vi "Registerkarten ein-ausblenden.vi"(0 "Registerkartenreferenz":refnum<vi>, 11 "error in (no error)":errorcluster caption="Fehler (Eingang, kein Fehler)", 13 "Aktion":T1) -> (15 "error out":errorcluster caption="Fehler (Ausgang)")   [LabVIEW 2020, in "EPA 1065.lvlib"]
uses:
  EPA 1065.lvlib
  Aktion Registerkarten ein-ausblenden.ctl
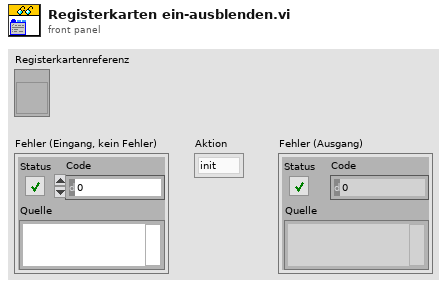
[diagram p1: front panel]
types:
  T1 = typedef "EPA 1065.lvlib/Aktion Registerkarten ein-ausblenden.ctl" = enum16{"init", "alle ausblenden", "Seite einblenden", "alle einblenden", "Seite deaktivieren", "Seiten aktivieren"}
  T2 = enum32{"Page Enabled", "Page Disabled", "Page Disabled & Grayed"}
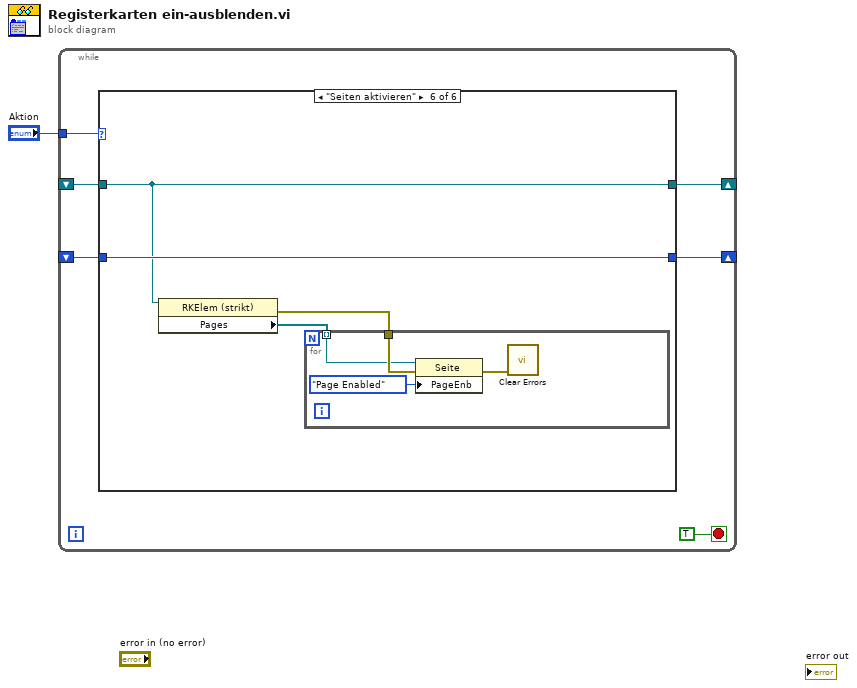
[diagram p0: block diagram]
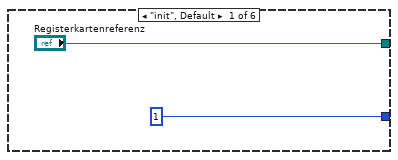
[diagram p2: hidden frame]
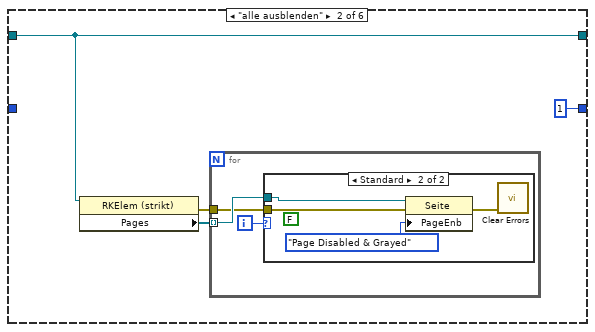
[diagram p3: hidden frame]
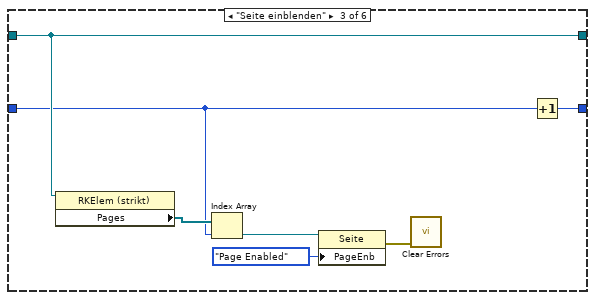
[diagram p5: hidden frame]
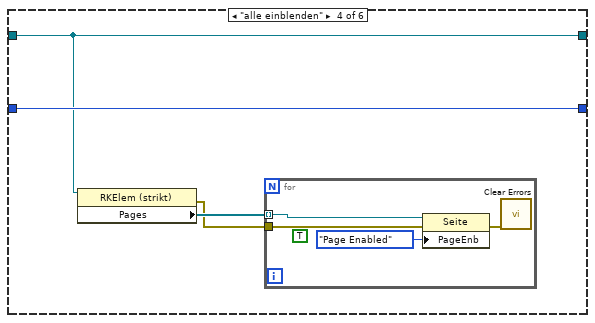
[diagram p6: hidden frame]
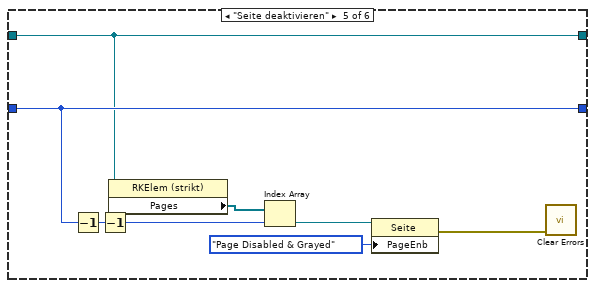
[diagram p7: hidden frame]
diagram:
  n1 = while {
    tunnel: "Aktion" -> [w7]
    shift-right: [w4] -> _
    shift-left: _ -> [w3]
    shift-right: [w5] -> _
    shift-left: _ -> [w2]
    stop <- TRUE stop-if-true
    n2 = case shown="\"Seiten aktivieren\"" w7 {
      tunnel: ["Registerkartenreferenz" w11 w26 w28 w38 w46] -> w5
      tunnel: [1 1 w27 w31 w43 w47] -> w4
      tunnel: w3 -> [_ _ w24 w31 w43 w47]
      tunnel: w2 -> [_ w11 w26 w28 w38 w46]
      frame "init", Default {
      }
      frame "alle ausblenden" {
        n3 = property class="RKElem (strikt)"(reference=w11) -> (error out=w12:errorcluster, "Pages"=w13:refnum<vi>[])  [unwired: 1 in, 1 out]
        n4 = for {
          tunnel: w13 -> [w16] mode=indexing
          tunnel: w12 -> [w14]
          i -> [w15]
          n5 = case shown="Standard" w15 {
            tunnel: w16 -> [_ w20]
            tunnel: w14 -> [_ w19]
            frame 0 {
            }
            frame Default {
              (unwired) FALSE ("Seite sichtbar")
              n6 = property class="Seite"(reference=w20, error in=w19, "PageEnb"=T2."Page Disabled & Grayed" ("Aktiv-Status der Seite")) -> (error out=w18:errorcluster)  [unwired: 1 out]
              n7 = call <vilib>:"Clear Errors.vi"("error in (no error)"=w18) -> ()  [unwired: 5 in, 2 out]
            }
          }
        }
      }
      frame "Seite einblenden" {
        n8 = property class="RKElem (strikt)"(reference=w26) -> ("Pages"=w25:refnum<vi>[])  [unwired: 1 in, 2 out]
        n9 = Index Array(array=w25, index=w24) -> (element=w21:refnum<vi>)
        n10 = property class="Seite"(reference=w21, "PageEnb"=T2."Page Enabled" ("Aktiv-Status der Seite")) -> (error out=w23:errorcluster)  [unwired: 1 in, 1 out]
        n11 = call <vilib>:"Clear Errors.vi"("error in (no error)"=w23) -> ()  [unwired: 5 in, 2 out]
        n12 = Increment(x=w24) -> (x+1=w27:i32)
      }
      frame "alle einblenden" {
        n13 = property class="RKElem (strikt)"(reference=w28) -> (error out=w29:errorcluster, "Pages"=w30:refnum<vi>[])  [unwired: 1 in, 1 out]
        n14 = for {
          tunnel: w30 -> [w35] mode=indexing
          tunnel: w29 -> [w34]
          (unwired) TRUE ("Seite sichtbar")
          n15 = property class="Seite"(reference=w35, error in=w34, "PageEnb"=T2."Page Enabled" ("Aktiv-Status der Seite")) -> (error out=w33:errorcluster)  [unwired: 1 out]
          n16 = call <vilib>:"Clear Errors.vi"("error in (no error)"=w33) -> ()  [unwired: 5 in, 2 out]
        }
      }
      frame "Seite deaktivieren" {
        n17 = Decrement(x=w43) -> (x-1=w37:i32)
        n18 = Decrement(x=w37) -> (x-1=w36:i32)
        n19 = property class="RKElem (strikt)"(reference=w38) -> ("Pages"=w42:refnum<vi>[])  [unwired: 1 in, 2 out]
        n20 = Index Array(array=w42, index=w36) -> (element=w40:refnum<vi>)
        n21 = property class="Seite"(reference=w40, "PageEnb"=T2."Page Disabled & Grayed" ("Aktiv-Status der Seite")) -> (error out=w41:errorcluster)  [unwired: 1 in, 1 out]
        n22 = call <vilib>:"Clear Errors.vi"("error in (no error)"=w41) -> ()  [unwired: 5 in, 2 out]
      }
      frame "Seiten aktivieren" {
        n23 = property class="RKElem (strikt)"(reference=w46) -> (error out=w44:errorcluster, "Pages"=w45:refnum<vi>[])  [unwired: 1 in, 1 out]
        n24 = for {
          tunnel: w45 -> [w48] mode=indexing
          tunnel: w44 -> [w49]
          n25 = property class="Seite"(reference=w48, error in=w49, "PageEnb"=T2."Page Enabled" ("Aktiv-Status der Seite")) -> (error out=w51:errorcluster)  [unwired: 1 out]
          n26 = call <vilib>:"Clear Errors.vi"("error in (no error)"=w51) -> ()  [unwired: 5 in, 2 out]
        }
      }
    }
  }
